vi "KeyenceCVX.Main.vi"() -> ()   [LabVIEW 2016]
uses:
  KeyenceCVX.Data.ctl
  KeyenceCVX.Data.Status.ctl
  KeyenceCVX.Data.Status.State.ctl
  KeyenceCVX.Data.Sets.ctl
  KeyenceCVX.CodeDetails.ctl
  KeyenceCVX.Action.ctl
  tools/CitTemplate/citTemplate.errData.ctl
  tools/EventLog/EventLog.EventSource.ctl
  private/controls/TriggerNo.ctl
  KeyenceCVX.ChangeProgram.Data.ctl
panel:
  out "Code":string
  out "Data out":T1
  out "_loop":i32(ring)=4
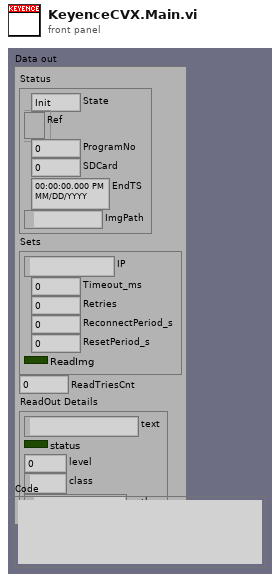
[diagram p1: front panel]
types:
  T1 = typedef "KeyenceCVX.Data.ctl" = cluster{"Status":T2, "Sets":T4, "ReadTriesCnt":u8, "ReadOut Details":T5}
  T2 = typedef "KeyenceCVX.Data.Status.ctl" = cluster{"State":T3, "Ref":refnum<k5>, "ProgramNo":u16, "SDCard":u8, "EndTS":timestamp, "ImgPath":path}
  T3 = typedef "KeyenceCVX.Data.Status.State.ctl" = enum16{"Init", "Reset", "Idle", "Scan"}
  T4 = typedef "KeyenceCVX.Data.Sets.ctl" = cluster{"IP":string, "Timeout_ms":i32, "Retries":i32, "ReconnectPeriod_s":i32, "ResetPeriod_s":i32, "ReadImg":bool}
  T5 = typedef "KeyenceCVX.CodeDetails.ctl" = cluster{"text":string, "status":bool, "level":u8, "class":string, "path":path}
  T6 = typedef "EventLog.EventSource.ctl" = enum16{"All", "Gui", "Ref", "File", "Arch", "Seq", "CPX", "DB", "Laser", "Scan.P", "Scan.O"}
  T7 = typedef "citTemplate.errData.ctl" = cluster{"ts":timestamp, "src":T6, "instance":i32, "action":string, "error":errorcluster, "unconfirmed":bool}
  T8 = typedef "KeyenceCVX.ChangeProgram.Data.ctl" = cluster{"SDCard":u8, "ProgramNo":u16}
  T9 = typedef "KeyenceCVX.Action.ctl" = enum32{"idle", "constructor", "destructor", "-- Keyence CVX --", "Init", "Scan", "ChangeProgram"}
  T10 = typedef "citTemplate.notifierHandle.ctl" = refnum<notifier>
  T11 = typedef "TriggerNo.ctl" = u8
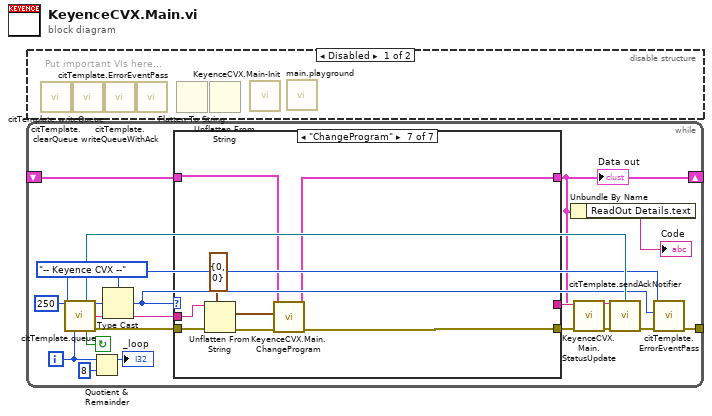
[diagram p0: block diagram]
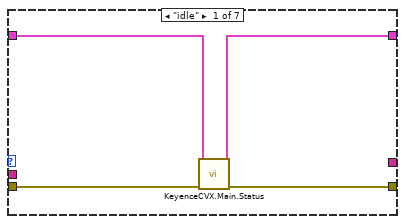
[diagram p3: hidden frame]
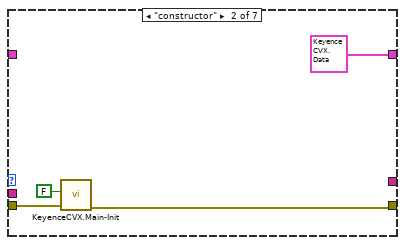
[diagram p4: hidden frame]
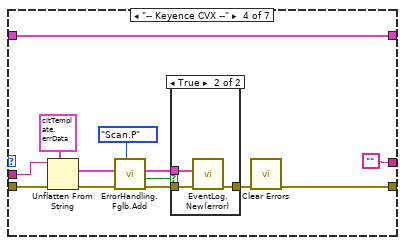
[diagram p6: hidden frame]
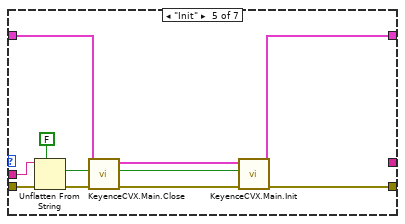
[diagram p8: hidden frame]
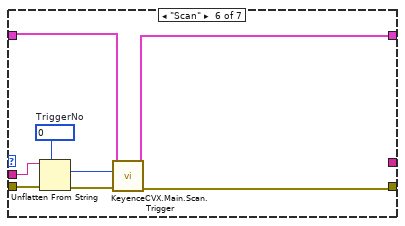
[diagram p9: hidden frame]
diagram:
  n1 = while {
    tunnel: [w9] -> _
    shift-right: [w1] -> _
    shift-left: _ -> [w4]
    i -> [w6]
    stop <- w15 continue-if-true
    w5 = KeyenceCVX.Action."-- Keyence CVX --" ("Action")
    n2 = call "citTemplate.queue.vi"("ms timeout (250 ms)"=250, "event enum"=w5, "iteration (-1)"=w6) -> ("notifierHandle out"=w14:T10, "event out"=w17:u32, "(flatten) data out"=w16:string, "continue"=w15:bool, "error out"=w7:errorcluster)  [unwired: 2 in, 6 out]
    n3 = Quotient & Remainder(x=w6, y=8) -> (x-y*floor(x/y)=→"_loop":i32)  [unwired: 1 out]
    n4 = Type Cast(type=w5, x=w17) -> (*(type *) &x=w10:T9)
    n5 = case shown="\"ChangeProgram\"" w10 {
      tunnel: w16 -> [_ _ _ w38 w48 w58 w68]
      tunnel: [_ _ _ "" _ _ _] -> w13
      tunnel: [w20 w24 w26 w30 w44 w55 w63] -> w2
      tunnel: [w18 T1 {"Status"={"State"=enum."Init", "Ref"=refnum, "ProgramNo"=0, "SDCard"=0, "EndTS"=timestamp(0 s since 1904-01-01), "ImgPath"=path ""}, "Sets"={"IP"="", "Timeout_ms"=0, "Retries"=0, "ReconnectPeriod_s"=0, "ResetPeriod_s"=0, "ReadImg"=FALSE}, "ReadTriesCnt"=0, "ReadOut Details"={"text"="", "status"=FALSE, "level"=0, "class"="", "path"=path ""}} ("Data out") w27 w28 w45 w54 w62] -> w1
      tunnel: w7 -> [w21 w25 w26 w37 w50 w60 w69]
      tunnel: w4 -> [w19 _ w27 w28 w52 w61 w66]
      frame "idle" {
        n6 = call "KeyenceCVX.Main.Status.vi"("error in"=w21, "Data"=w19) -> ("error out"=w20:errorcluster, "Data out"=w18:T1)  [unwired: 8 in]
      }
      frame "constructor" {
        n7 = call "KeyenceCVX.Main-Init.vi"("error in"=w25, "restart (T)"=FALSE) -> ("error out"=w24:errorcluster)  [unwired: 9 in]
      }
      frame "destructor" {
      }
      frame "-- Keyence CVX --" {
        n8 = Unflatten From String(type=T7 {"ts"=timestamp(0 s since 1904-01-01), "src"=enum."All", "instance"=0, "action"="", "error"={"status"=FALSE, "code"=0, "source"=""}, "unconfirmed"=FALSE} ("ErrData"), binary string=w38, error in (no error)=w37) -> (value=w33:T7, error out=w32:errorcluster)  [unwired: 3 out]
        n9 = call "ErrorHandling.Fglb.Add.vi"("Event source"=EventLog.EventSource."Scan.P", "error in (no error)"=w32, "Error in"=w33) -> ("error out"=w35:errorcluster, "changed?"=w31:bool)  [unwired: 7 in]
        n10 = case shown="True" w31 {
          tunnel: w35 -> [w40 w43]
          tunnel: [w40 w42] -> w34
          tunnel: w33 -> [_ w41]
          frame False {
          }
          frame True {
            n11 = call "EventLog.New(error).vi"("error in"=w43, "ErrData"=w41) -> ("error out"=w42:errorcluster)  [unwired: 9 in]
          }
        }
        n12 = call <vilib>:"Clear Errors.vi"("error in (no error)"=w34) -> ("error out"=w30:errorcluster)  [unwired: 5 in, 1 out]
      }
      frame "Init" {
        n13 = Unflatten From String(type=FALSE, binary string=w48, error in (no error)=w50) -> (value=w46:bool, error out=w49:errorcluster)  [unwired: 2 in, 1 out]
        n14 = call "KeyenceCVX.Main.Close.vi"("error in"=w49, "Data in"=w52) -> ("error out"=w53:errorcluster, "Data out"=w51:T1)  [unwired: 8 in]
        n15 = call "KeyenceCVX.Main.Init.vi"("error in"=w53, "restart"=w46, "Data"=w51) -> ("error out"=w44:errorcluster, "Data out"=w45:T1)  [unwired: 7 in]
      }
      frame "Scan" {
        w59 = T11 0 items=["1"=1, "2"=2, "3"=3, "4"=4, "ALL"=5]  # TriggerNo
        n16 = Unflatten From String(type=w59, binary string=w58, error in (no error)=w60) -> (value=w57:T11, error out=w56:errorcluster)  [unwired: 2 in, 1 out]
        n17 = call "KeyenceCVX.Main.Scan.Trigger.vi"("error in"=w56, "TriggerNo"=w57, "Data"=w61) -> ("error out"=w55:errorcluster, "Data out"=w54:T1)  [unwired: 7 in]
      }
      frame "ChangeProgram" {
        n18 = Unflatten From String(type=T8 {"SDCard"=0, "ProgramNo"=0} ("ChangeProgram.Data"), binary string=w68, error in (no error)=w69) -> (value=w65:T8, error out=w64:errorcluster)  [unwired: 2 in, 1 out]
        n19 = call "KeyenceCVX.Main.ChangeProgram.vi"("error in"=w64, "ChangeProgram.Data"=w65, "Data"=w66) -> ("error out"=w63:errorcluster, "Data out"=w62:T1)  [unwired: 7 in]
      }
    }
    "Data out" <- w1
    n20 = Unbundle By Name(w1) -> ("ReadOut Details.text"=→"Code":string)
    n21 = call "KeyenceCVX.Main.StatusUpdate.vi"("error in"=w2, "Data in"=w1) -> ()  [unwired: 9 in, 1 out]
    n22 = call "citTemplate.sendAckNotifier.vi"("notification data"=w13, "notifierHandle in"=w14, "error in"=w2) -> ()  [unwired: 13 out]
    n23 = call "citTemplate.ErrorEventPass.vi"("error in"=w2, "action of error"=w10, "event in"=w5) -> ("error out"=w9:errorcluster)  [unwired: 2 in, 6 out]
  }
  n24 = disable-structure shown="Disabled" {
    frame Disabled {
      # "Put important VIs here..."
      n25 = call "citTemplate.clearQueue.vi"() -> ()  [unwired: 14 in, 2 out]
      n26 = call "citTemplate.writeQueue.vi"() -> ()  [unwired: 15 in, 1 out]
      n27 = call "citTemplate.writeQueueWithAck.vi"() -> ()  [unwired: 13 in, 3 out]
      n28 = call "citTemplate.ErrorEventPass.vi"() -> ()  [unwired: 11 in, 1 out]
      n29 = Flatten To String() -> ()  [unwired: 4 in, 3 out]
      n30 = Unflatten From String() -> ()  [unwired: 5 in, 3 out]
      n31 = call "KeyenceCVX.Main-Init.vi"() -> ()  [unwired: 11 in, 1 out]
      n32 = call "main.playground.vi"() -> ()  [unwired: 12 in]
    }
    frame Enabled {
    }
  }
